vi "HLG Send Email.vi"(1 "Body":string="Helium Level Report", 2 "CC - Optional":string, 4 "Recipient's Email Address":string="phyzrx@gmail.com") -> ()   [LabVIEW 2014]
panel:
  in  "Attachment - Optional":path
  in  "Port":i32=587
  in  "Enable SSL":bool=TRUE
  in  "GMAIL Account Password":string="Uz&A=6U]w^"
  in  "GMAIL Account User ID":string="hlg.penn.state@gmail.com"
  in  "Outgoing Mail Server (SMTP)":string="smtp.gmail.com"
  in  "Subject":string="Helium Level Report"
  in  "Recipient's Name":string="Helium Level"
  in  "Sender's Name":string="Helium Level"
  in  "Sender's Email Address (eg: LabVIEW@gmail.com)":string="hlg.penn.state@gmail.com"
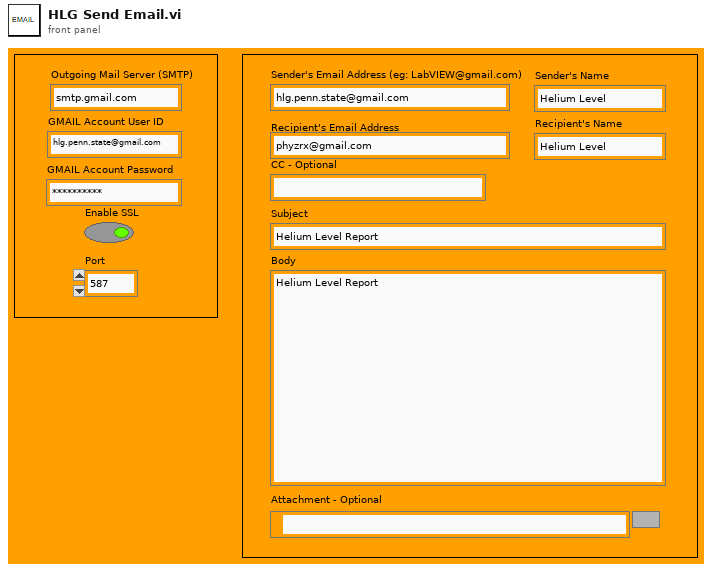
[diagram p1: front panel]
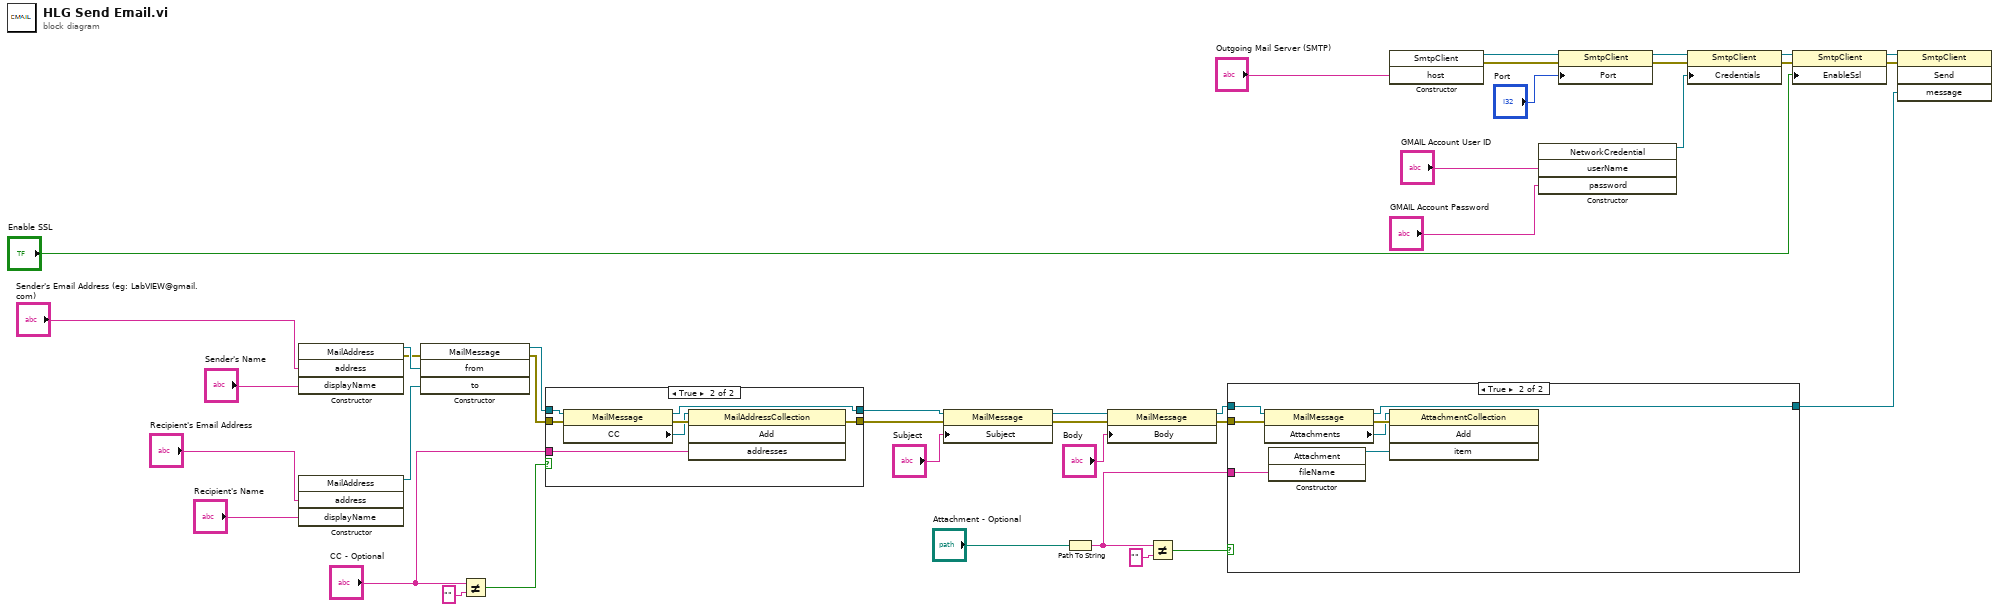
[diagram p0: block diagram]
diagram:
  n1 = constructor class="MailAddress"("address"="Sender's Email Address (eg: LabVIEW@gmail.com)", "displayName"="Sender's Name") -> (reference out=w38:refnum<k24>, error out=w2:errorcluster)  [unwired: 3 in, 3 out]
  n2 = constructor class="MailAddress"("address"="Recipient's Email Address", "displayName"="Recipient's Name") -> (reference out=w39:refnum<k24>)  [unwired: 3 in, 4 out]
  n3 = constructor class="MailMessage"(error in=w2, "from"=w38, "to"=w39) -> (reference out=w9:refnum<k24>, error out=w8:errorcluster)  [unwired: 2 in, 3 out]
  n4 = Not Equal?(x="CC - Optional", y="") -> (x != y?=w11:bool)
  n5 = case shown="True" w11 {
    tunnel: "CC - Optional" -> [_ w46]
    tunnel: w9 -> [w41 w45]
    tunnel: w8 -> [w40 w44]
    tunnel: [w41 w43] -> w7
    tunnel: [w40 w42] -> w6
    frame False {
    }
    frame True {
      n6 = property class="MailMessage"(reference=w45, error in=w44) -> (reference out=w43:refnum<k24>, error out=w48:errorcluster, "CC"=w47:refnum<k24>)
      n7 = invoke class="MailAddressCollection" method="Add"(reference=w47, error in=w48, "addresses"=w46) -> (error out=w42:errorcluster)  [unwired: 1 in, 3 out]
    }
  }
  n8 = property class="MailMessage"(reference=w7, error in=w6, "Subject"="Subject") -> (reference out=w29:refnum<k24>, error out=w37:errorcluster)
  n9 = Path To String(path="Attachment - Optional") -> (string=w13:string)
  n10 = property class="MailMessage"(reference=w29, error in=w37, "Body"="Body") -> (reference out=w17:refnum<k24>, error out=w1:errorcluster)
  n11 = Not Equal?(x=w13, y="") -> (x != y?=w14:bool)
  n12 = case shown="True" w14 {
    tunnel: w17 -> [w49 w53]
    tunnel: [w49 w52] -> w5
    tunnel: w13 -> [_ w51]
    tunnel: w1 -> [_ w50]
    frame False {
    }
    frame True {
      n13 = property class="MailMessage"(reference=w53, error in=w50) -> (reference out=w52:refnum<k24>, error out=w56:errorcluster, "Attachments"=w54:refnum<k24>)
      n14 = constructor class="Attachment"("fileName"=w51) -> (reference out=w55:refnum<k24>)  [unwired: 3 in, 3 out]
      n15 = invoke class="AttachmentCollection" method="Add"(reference=w54, error in=w56, "item"=w55) -> ()  [unwired: 1 in, 4 out]
    }
  }
  n16 = constructor class="SmtpClient"("host"="Outgoing Mail Server (SMTP)") -> (reference out=w23:refnum<k24>, error out=w20:errorcluster)  [unwired: 3 in, 2 out]
  n17 = constructor class="NetworkCredential"("userName"="GMAIL Account User ID", "password"="GMAIL Account Password") -> (reference out=w24:refnum<k24>)  [unwired: 3 in, 4 out]
  n18 = property class="SmtpClient"(reference=w23, error in=w20, "Port"="Port") -> (reference out=w22:refnum<k24>, error out=w19:errorcluster)
  n19 = property class="SmtpClient"(reference=w22, error in=w19, "Credentials"=w24) -> (reference out=w21:refnum<k24>, error out=w18:errorcluster)
  n20 = property class="SmtpClient"(reference=w21, error in=w18, "EnableSsl"="Enable SSL") -> (reference out=w3:refnum<k24>, error out=w4:errorcluster)
  n21 = invoke class="SmtpClient" method="Send"(reference=w3, error in=w4, "message"=w5) -> ()  [unwired: 1 in, 4 out]
